vi "Dynamic Call__Uti.vi"(8 "error in (no error)":errorcluster, 10 "open front panel? (T)":bool=TRUE, 11 "vi path":path) -> (0 "error out":errorcluster)   [LabVIEW 2012]
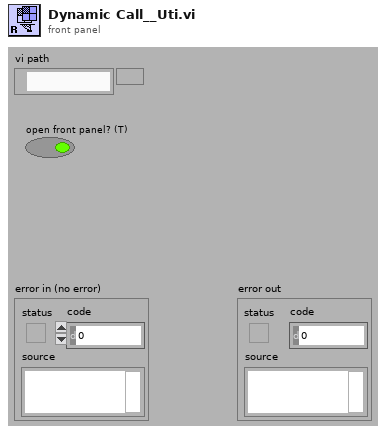
[diagram p1: front panel]
types:
  T1 = enum32{"Bad", "Idle", "Run top level", "Running"}
  T2 = enum32{"Invalid", "Standard", "Closed", "Hidden", "Minimized", "Maximized"}
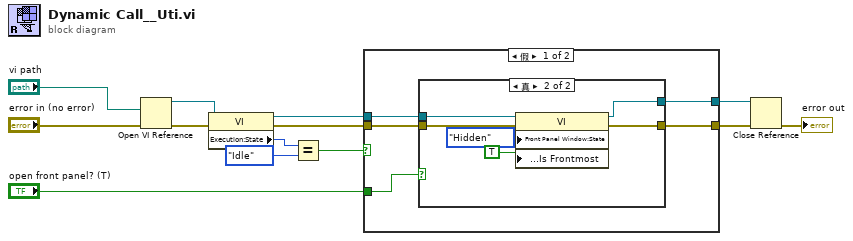
[diagram p0: block diagram]
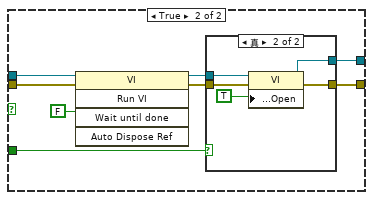
[diagram p3: hidden frame]
diagram:
  n1 = Open VI Reference(vi path="vi path", error in (no error)="error in (no error)") -> (vi reference=w6:refnum<vi>, error out=w4:errorcluster)  [unwired: 4 in]
  n2 = property class="VI"(reference=w6, error in=w4) -> (reference out=w5:refnum<vi>, error out=w2:errorcluster, "Execution:State"=w8:T1)
  n3 = Equal?(x=w8, y=T1."Idle") -> (x = y?=w3:bool)
  n4 = case shown="假" w3 {
    tunnel: [w15 w31] -> w10
    tunnel: [w16 w30] -> w9
    tunnel: w5 -> [w18 w29]
    tunnel: w2 -> [w17 w28]
    tunnel: "open front panel? (T)" -> [w14 w27]
    frame False {
      n5 = case shown="真" w14 {
        tunnel: w18 -> [w20 w26]
        tunnel: w17 -> [w19 w25]
        tunnel: [w19 w24] -> w16
        tunnel: [w20 w23] -> w15
        frame False {
        }
        frame True {
          n6 = property class="VI"(reference=w26, error in=w25, "Front Panel Window:State"=T2."Hidden", "Front Panel Window:Is Frontmost"=TRUE) -> (reference out=w23:refnum<vi>, error out=w24:errorcluster)
        }
      }
    }
    frame True {
      n7 = invoke class="VI" method="Run VI"(reference=w29, error in=w28, "Wait until done"=FALSE) -> (reference out=w32:refnum<vi>, error out=w33:errorcluster)  [unwired: 2 in, 3 out]
      n8 = case shown="真" w27 {
        tunnel: w33 -> [w35 w40]
        tunnel: w32 -> [w36 w39]
        tunnel: [w36 w38] -> w31
        tunnel: [w35 w37] -> w30
        frame False {
        }
        frame True {
          n9 = property class="VI"(reference=w39, error in=w40, "Front Panel Window:Open"=TRUE) -> (reference out=w38:refnum<vi>, error out=w37:errorcluster)
        }
      }
    }
  }
  n10 = Close Reference(reference=w10, error in (no error)=w9) -> (error out=→"error out":errorcluster)
